vi "v0.2_son_serial.vi"(8 "error in (no error)":errorcluster, 10 "ServoON":bool, 11 "VISA COM IN":refnum<visa-resource-name>) -> (0 "error out":errorcluster, 3 "VISA COM OUT":refnum<visa-resource-name>)   [LabVIEW 2011]
doc: "<B>Servo ON</B>\n\nEncender/Apagar el servomotor utilizando una variable boolena"
panel:
  # "Enciende o Apaga el Servomotor"
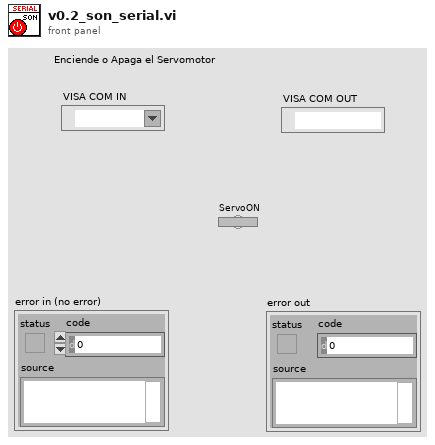
[diagram p1: front panel]
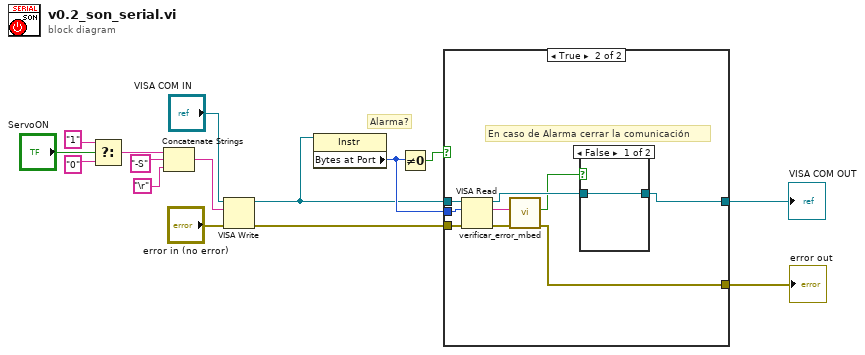
[diagram p0: block diagram]
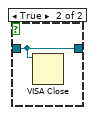
[diagram p3: hidden frame]
diagram:
  # "Alarma?"
  n1 = Select(t="1" ("string"), s="ServoON", f="0" ("string")) -> (s? t:f=w8:string)
  n2 = Concatenate Strings(w8, "-S" ("string"), "\r") -> (w13:string)
  n3 = VISA Write(VISA resource name="VISA COM IN", write buffer=w13, error in (no error)="error in (no error)") -> (VISA resource name out=w4:refnum<visa-resource-name>, error out=w3:errorcluster)  [unwired: 1 out]
  n4 = property class="Instr"(reference=w4) -> ("Bytes at Port"=w5:u32)  [unwired: 1 in, 2 out]
  n5 = Not Equal To 0?(x=w5) -> (x != 0?=w6:bool)
  n6 = case shown="True" w6 {
    tunnel: w4 -> [w17 w23]
    tunnel: w3 -> [w16 w22]
    tunnel: w5 -> [_ w20]
    tunnel: [w17 w19] -> w2
    tunnel: [w16 w18] -> w1
    frame False {
    }
    frame True {
      # "En caso de Alarma cerrar la comunicación"
      n7 = VISA Read(VISA resource name=w23, byte count=w20, error in (no error)=w22) -> (VISA resource name out=w24:refnum<visa-resource-name>, read buffer=w25:string, error out=w26:errorcluster)  [unwired: 1 out]
      n8 = call "verificar_error_mbed.vi"("error in (no error)"=w26, "desde_mbed"=w25) -> ("error out"=w18:errorcluster, "error?"=w21:bool)  [unwired: 8 in]
      n9 = case shown="False" w21 {
        tunnel: w24 -> [w27 w28]
        tunnel: [w27 w28] -> w19
        frame False {
        }
        frame True {
          n10 = VISA Close(VISA resource name=w28) -> ()  [unwired: 1 in, 1 out]
        }
      }
    }
  }
  "VISA COM OUT" <- w2
  "error out" <- w1
